vi "Test Assert Equal Value.vi"(8 "error in (no error)":errorcluster) -> (0 "error out":errorcluster)   [LabVIEW 2009]
uses:
  classes/Assert/Assert.lvclass
  classes/Test/Test.lvclass
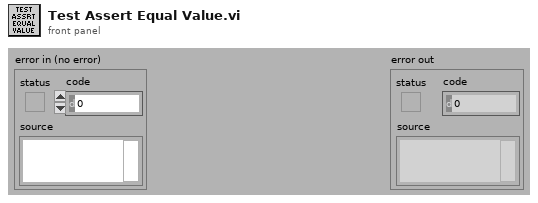
[diagram p1: front panel]
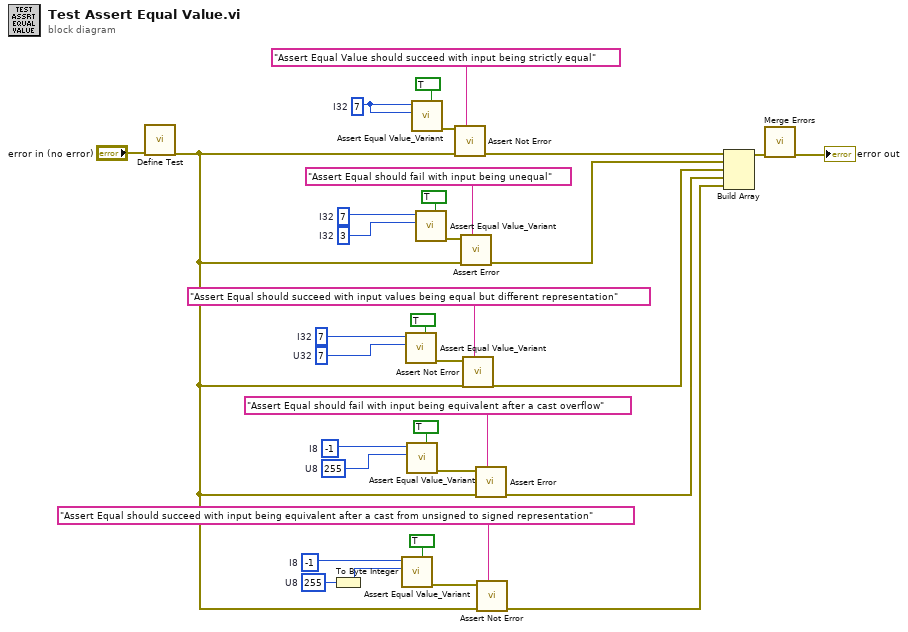
[diagram p0: block diagram]
diagram:
  w16 = 3  # I32
  w17 = 7  # I32
  w22 = 7  # I32
  w26 = u8 255  # U8
  w6 = i8 -1  # I8
  w8 = u8 255  # U8
  w9 = i8 -1  # I8
  w2 = u32 7  # U32
  w3 = 7  # I32
  n1 = call "Define Test.vi"("error in (no error)"="error in (no error)") -> ("error out"=w1:errorcluster)  [unwired: 10 in]
  n2 = To Byte Integer(number=w26) -> (8bit integer=w5:i8)
  n3 = call "Assert Equal Value_Variant.vi"("Assert Only? (F)"=TRUE, "Y"=w5, "X"=w6) -> ("error out"=w4:errorcluster)  [unwired: 8 in]
  n4 = call "Assert Equal Value_Variant.vi"("Assert Only? (F)"=TRUE, "Y"=w2, "X"=w3) -> ("error out"=w14:errorcluster)  [unwired: 8 in]
  n5 = call "Assert Equal Value_Variant.vi"("Assert Only? (F)"=TRUE, "Y"=w8, "X"=w9) -> ("error out"=w11:errorcluster)  [unwired: 8 in]
  n6 = call "Assert Equal Value_Variant.vi"("Assert Only? (F)"=TRUE, "Y"=w22, "X"=w22) -> ("error out"=w21:errorcluster)  [unwired: 8 in]
  n7 = call "Assert Equal Value_Variant.vi"("Assert Only? (F)"=TRUE, "Y"=w16, "X"=w17) -> ("error out"=w20:errorcluster)  [unwired: 8 in]
  n8 = call "Assert Not Error.vi"("Label"="Assert Equal Value should succeed with input being strictly equal", "error in (no error)"=w1, "Not Error?"=w21) -> ("error out"=w30:errorcluster)  [unwired: 8 in]
  n9 = call "Assert Error.vi"("Label"="Assert Equal should fail with input being unequal", "error in (no error)"=w1, "Error?"=w20) -> ("error out"=w29:errorcluster)  [unwired: 8 in]
  n10 = call "Assert Not Error.vi"("Label"="Assert Equal should succeed with input values being equal but different representation", "error in (no error)"=w1, "Not Error?"=w14) -> ("error out"=w13:errorcluster)  [unwired: 8 in]
  n11 = call "Assert Error.vi"("Label"="Assert Equal should fail with input being equivalent after a cast overflow", "error in (no error)"=w1, "Error?"=w11) -> ("error out"=w24:errorcluster)  [unwired: 8 in]
  n12 = call "Assert Not Error.vi"("Label"="Assert Equal should succeed with input being equivalent after a cast from unsigned to signed representation", "error in (no error)"=w1, "Not Error?"=w4) -> ("error out"=w23:errorcluster)  [unwired: 8 in]
  n13 = Build Array(w30, w29, w13, w24, w23) -> (w28:errorcluster[])
  n14 = call <vilib>:"Merge Errors.vi"("error array in"=w28) -> ("error out"=→"error out":errorcluster)  [unwired: 6 in]
